vi "SLL DE AO Safe Values LV2 Global.vi"(7 "Cases":T2, 8 "error in (no error)":errorcluster, 10 "Value In":dbl[](array[numeric]), 11 "Elements In":T1[](array[typedef])) -> (0 "error out":errorcluster, 2 "Value Array Out":dbl[](array[numeric]), 3 "Elements Out":T1[](array[typedef]))   [LabVIEW 2009]
uses:
  Controls/SLL DE AO Safe Value Global Options.ctl
  Controls/SLL DE List of Analog Outputs.ctl
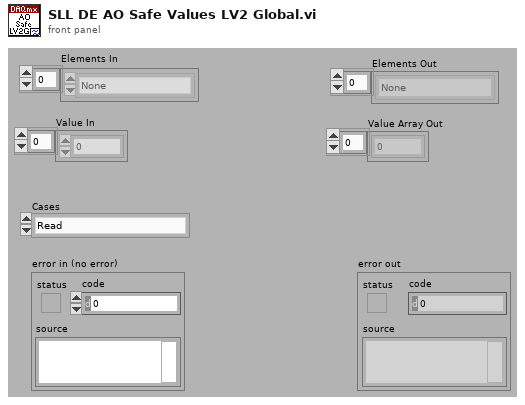
[diagram p1: front panel]
types:
  T1 = typedef "SLL DE List of Analog Outputs.ctl" = enum16{"None"}
  T2 = typedef "SLL DE AO Safe Value Global Options.ctl" = enum16{"Read", "Write"}
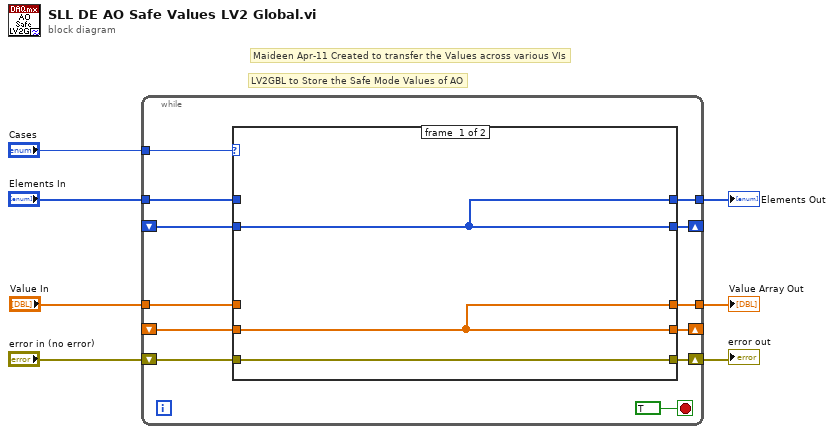
[diagram p0: block diagram]
diagram:
  # "Maideen Apr-11 Created to transfer the Values across various VIs"
  # "LV2GBL to Store the Safe Mode Values of AO"
  n1 = while {
    shift-right: [w18] -> _
    shift-left: _ -> [w17]
    tunnel: "Elements In" -> [w16]
    tunnel: [w15] -> w6
    shift-right: [w13] -> w4
    shift-left: "error in (no error)" -> [w14]
    tunnel: "Value In" -> [w12]
    tunnel: "Cases" -> [w11]
    tunnel: [w10] -> w1
    shift-right: [w9] -> _
    shift-left: _ -> [w8]
    stop <- TRUE stop-if-true
    n2 = case shown="\"Read\", Default" w11 {
      tunnel: [w21 w25] -> w18
      tunnel: w17 -> [w21 _]
      tunnel: w16 -> [_ w24]
      tunnel: [w21 w25] -> w15
      tunnel: w14 -> [w22 w23]
      tunnel: [w22 w23] -> w13
      tunnel: w12 -> [_ w25]
      tunnel: [w20 w24] -> w10
      tunnel: [w20 w24] -> w9
      tunnel: w8 -> [w20 _]
      frame #0 {
      }
      frame #1 {
      }
    }
  }
  "error out" <- w4
  "Value Array Out" <- w6
  "Elements Out" <- w1
